vi "SetPreviousData.vi"(6 "Cancel pipe? (F)":bool, 8 "error in (no error)":errorcluster, 10 "Data":variant, 11 "SMP in":refnum<class "SMP.lvclass">) -> (0 "error out":errorcluster, 3 "SMP out":refnum<class "SMP.lvclass">)   [LabVIEW 2013, in "SMP.lvclass"]
doc: "Sets the data which was produced by the last operation and which should be available for the next operation in the queue. This data will be provided via the \"Previous data\" terminal of the GetOperation function, when the next operation is retrieved from the internal queue.\n\nThis function executes even if there is an error on its \"error in\" terminal.\n\n<b>Cancel pipe: </b>Wire TRUE to cancel any remaining operation in the current pipe. This input is ignored if there is no pipe currently in execution. Default is FALSE."
uses:
  SMP.lvclass
  Data types/operation.ctl
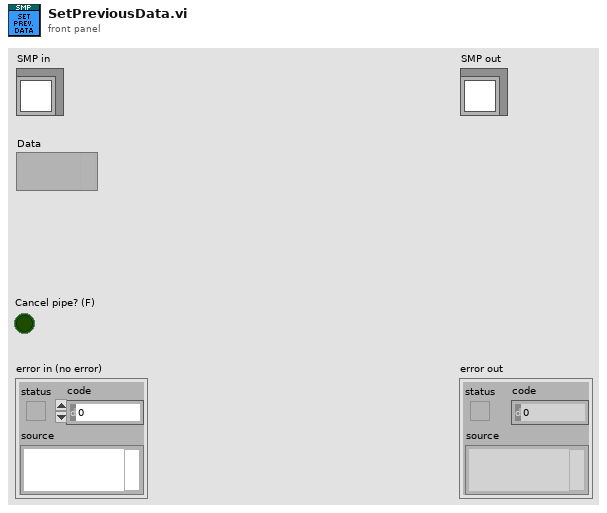
[diagram p1: front panel]
types:
  T1 = typedef "SMP.lvclass/operation.ctl" = cluster{"Name":string, "Data":variant}
  T2 = typedef "Pipe and Filter.lvclass/classData.ctl" = cluster{"Q ref":refnum<queue>, "Previous data":variant, "Current pipe":T3[]}
  T3 = typedef "Pipe and Filter.lvclass/operation.ctl" = cluster{"Name":string, "Data":variant}
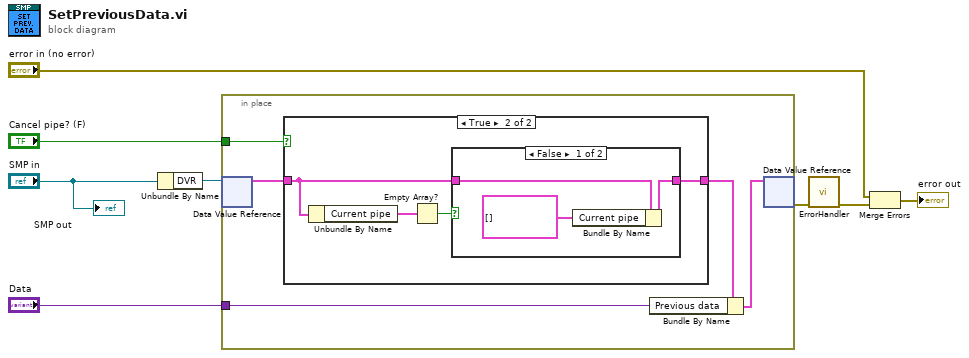
[diagram p0: block diagram]
diagram:
  n1 = Unbundle By Name("SMP in") -> ("DVR"=w4:refnum<data-value>)
  n2 = in-place {
    in-place-border: "Cancel pipe? (F)" -> [w12]
    in-place-border: "Data" -> [w9]
    n3 = in-place-dvr #1(w4) -> (w13:T2)  [unwired: 1 out]
    n4 = case shown="True" w12 {
      tunnel: w13 -> [w14 w16]
      tunnel: [w14 w15] -> w11
      frame False {
      }
      frame True {
        n5 = Unbundle By Name(w16) -> ("Current pipe"=w17:T3[])
        n6 = Empty Array?(array=w17) -> (empty?=w18:bool)
        n7 = case shown="False" w18 {
          tunnel: w16 -> [w21 w22]
          tunnel: [w20 w22] -> w15
          frame False {
            n8 = Bundle By Name(cluster=w21, "Current pipe"=T1[] []) -> (w20:T2)
          }
          frame True {
          }
        }
      }
    }
    n9 = Bundle By Name(cluster=w11, "Previous data"=w9) -> (w10:T2)
    n10 = in-place-dvr #1(w10) -> (w3:errorcluster)  [unwired: 1 out]
  }
  n11 = call "ErrorHandler.vi"("error in (no error)"=w3) -> ("error out"=w8:errorcluster)  [unwired: 9 in, 1 out]
  n12 = Merge Errors("error in (no error)", w8) -> (→"error out":errorcluster)
  "SMP out" <- "SMP in"
